vi "bigcryo_H-full_ver2.vi"() -> ()   [LabVIEW 2019]
uses:
  B_Globals.vi
  <vilib>/Analysis/NI_AALPro.lvlib
panel:
  out "Stable":bool
  out "Act. Rate [T/min]":dbl
  out "Read Buffer":string="0"
  in  "stop":bool
  out "Its":i32
  out "Running Sequence":bool
  in  "Set Field":dbl
  in  "Rate":dbl=0.2
  in  "Go To":bool=TRUE
  out "Field [T]":dbl=10.348
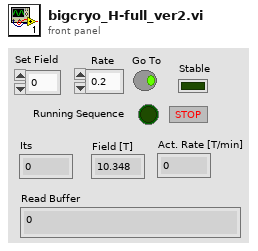
[diagram p1: front panel]
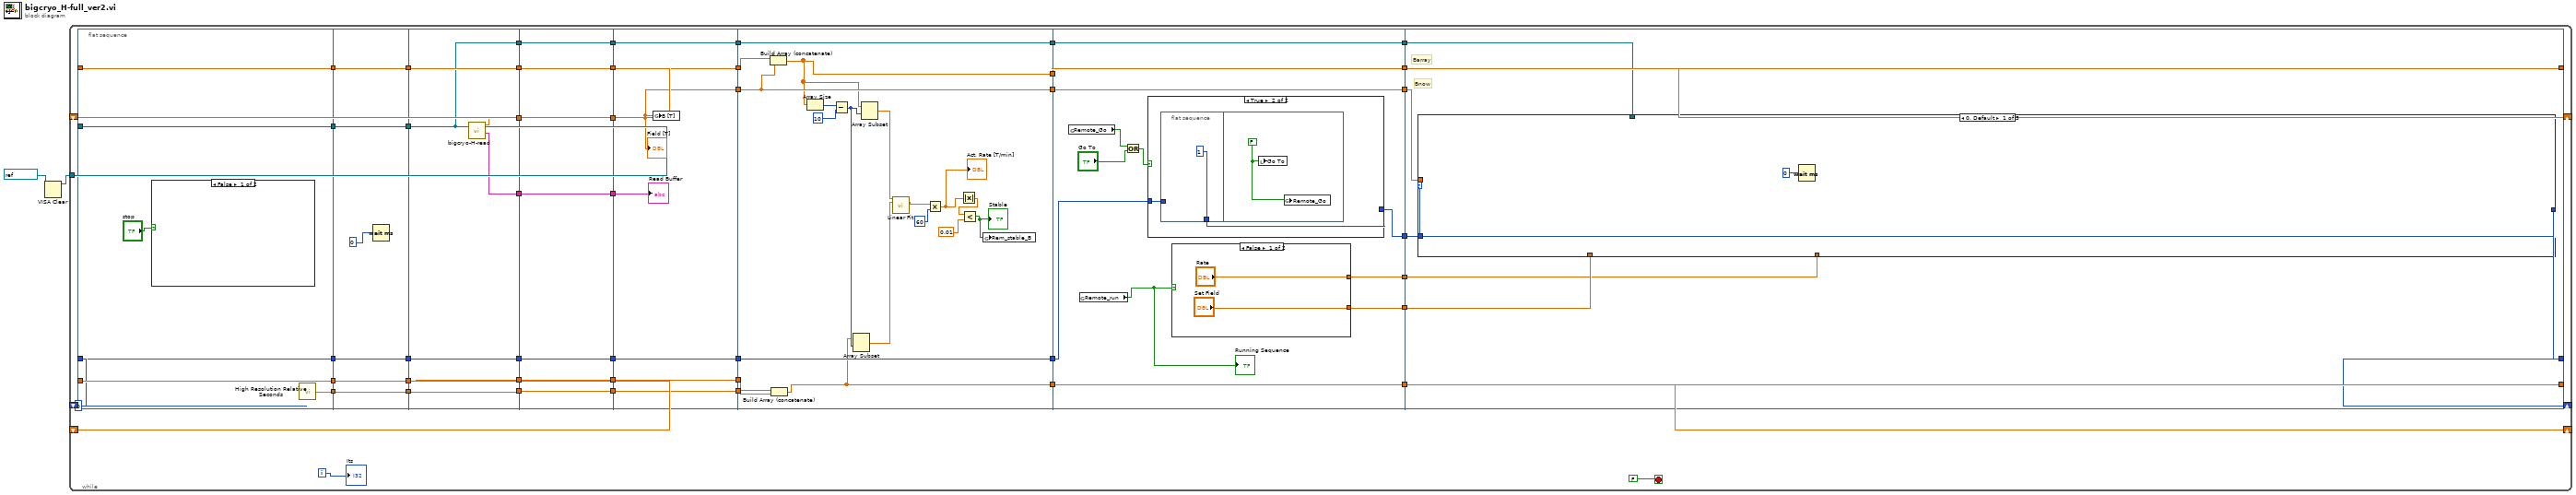
[diagram p0: block diagram]
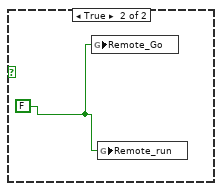
[diagram p2: hidden frame]
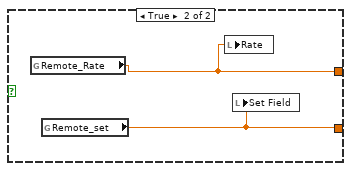
[diagram p3: hidden frame]
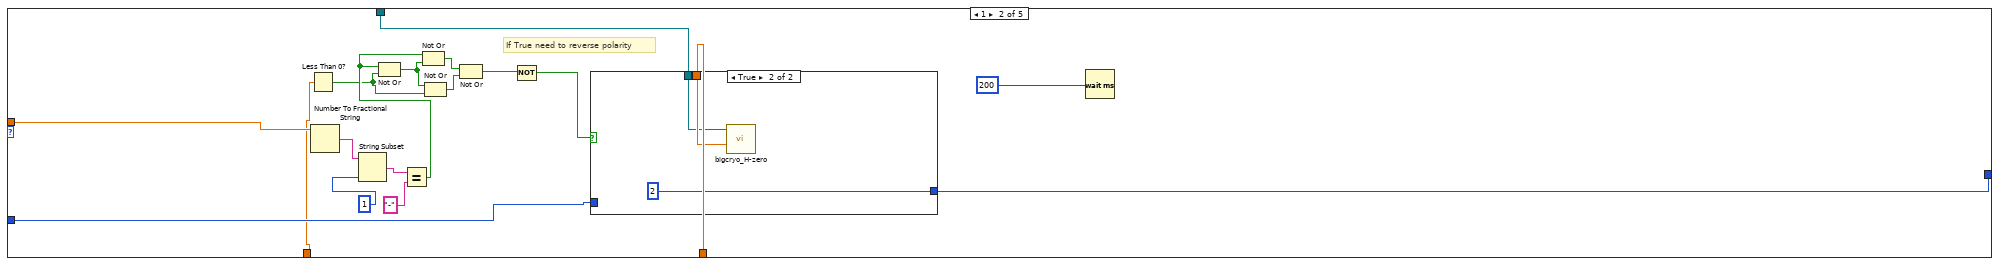
[diagram p5: hidden frame]
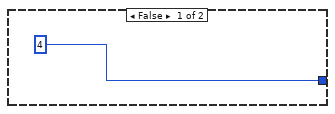
[diagram p6: hidden frame]
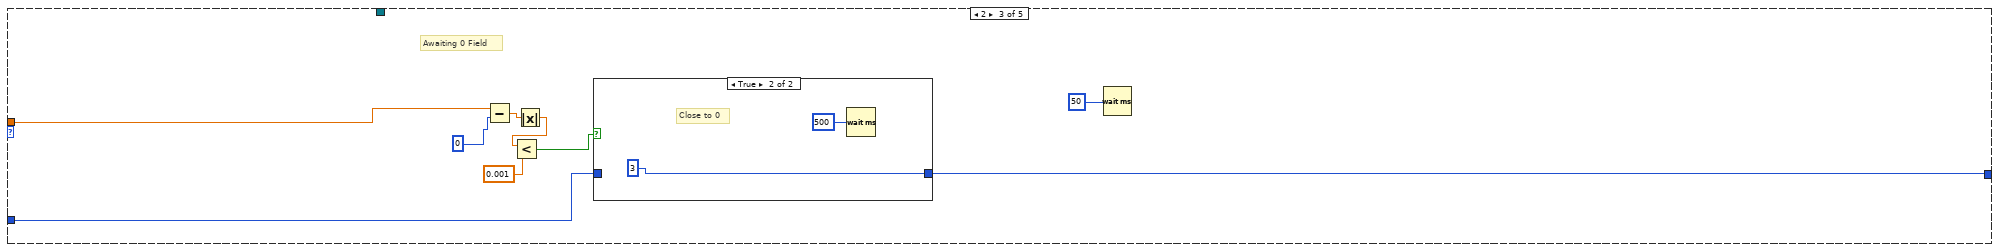
[diagram p7: hidden frame]
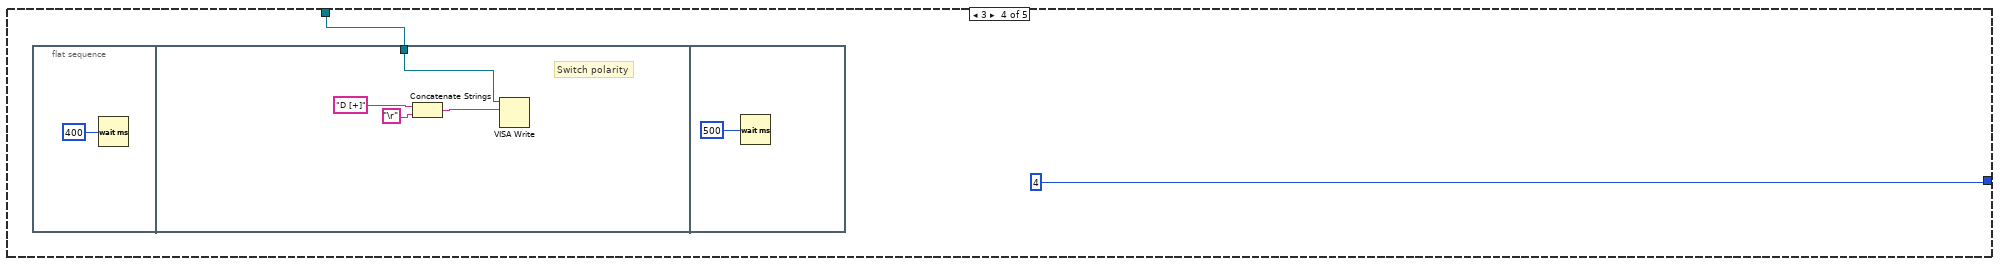
[diagram p9: hidden frame]
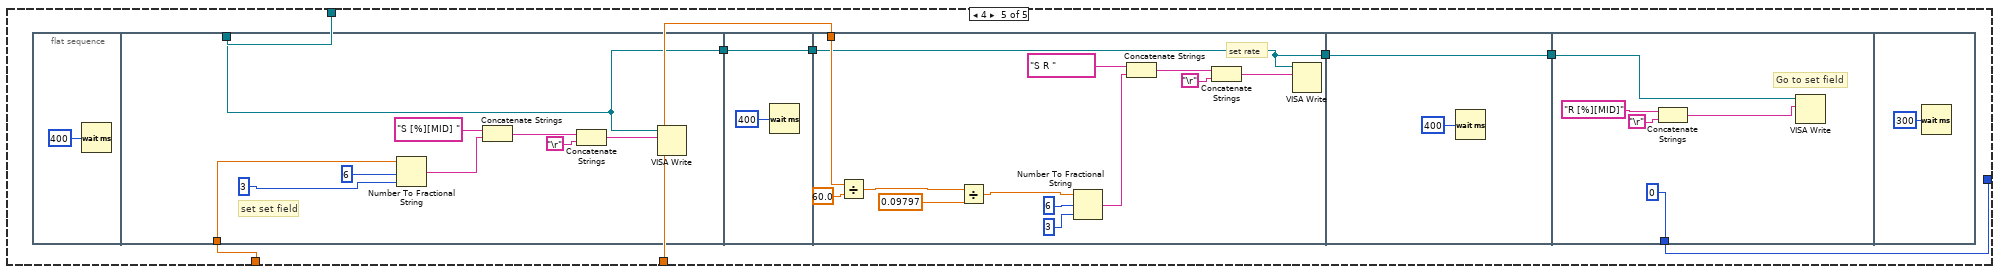
[diagram p10: hidden frame]
diagram:
  n1 = VISA Clear(VISA resource name=refnum<visa-resource-name> "COM6" ("Lakeshore Address")) -> (VISA resource name out=w2:refnum<visa-resource-name>)  [unwired: 1 in, 1 out]
  n2 = while {
    shift-right: [w52] -> _
    shift-left: _ -> [w53]
    shift-right: [w49] -> _
    shift-left: _ -> [w50]
    tunnel: w2 -> [w54]
    shift-right: [w40] -> _
    shift-left: 0 -> [w46]
    i -> [w31]
    stop <- FALSE stop-if-true
    n3 = flat-sequence {
      tunnel: w46 -> [w57]
      tunnel: w50 -> [w58]
      tunnel: w53 -> [w59]
      tunnel: w54 -> [w60]
      tunnel: [w60] -> w13
      tunnel: [w59] -> w11
      tunnel: [w58] -> w9
      tunnel: [w57] -> w7
      tunnel: [w55] -> w5
      tunnel: w13 -> [w67]
      tunnel: [w67] -> w12
      tunnel: w11 -> [w66]
      tunnel: [w66] -> w10
      tunnel: w9 -> [w65]
      tunnel: [w65] -> w8
      tunnel: w7 -> [w64]
      tunnel: [w64] -> w6
      tunnel: w5 -> [w63]
      tunnel: [w63] -> w4
      tunnel: [w74] -> w30
      tunnel: [w73] -> w28
      tunnel: [w72] -> w26
      tunnel: [w68] -> w24
      tunnel: [w71] -> w22
      tunnel: [w70] -> w20
      tunnel: w12 -> [w70]
      tunnel: w10 -> [w73]
      tunnel: w8 -> [w72]
      tunnel: w6 -> [w71]
      tunnel: [w69] -> w18
      tunnel: w4 -> [w68]
      tunnel: w30 -> [w81]
      tunnel: [w81] -> w29
      tunnel: w28 -> [w80]
      tunnel: [w80] -> w27
      tunnel: w26 -> [w79]
      tunnel: [w79] -> w25
      tunnel: w24 -> [w78]
      tunnel: [w78] -> w23
      tunnel: w22 -> [w77]
      tunnel: [w77] -> w21
      tunnel: w20 -> [w76]
      tunnel: [w76] -> w19
      tunnel: w18 -> [w75]
      tunnel: [w75] -> w17
      tunnel: w29 -> [w82]
      tunnel: w27 -> [w83]
      tunnel: w25 -> [w85]
      tunnel: w23 -> [w84]
      tunnel: w21 -> [w88]
      tunnel: [w88] -> w44
      tunnel: [w82] -> w37
      tunnel: w19 -> [w87]
      tunnel: [w87] -> w35
      tunnel: w17 -> [w86]
      tunnel: [w85] -> w16
      tunnel: [w84] -> w15
      tunnel: [w83] -> w14
      tunnel: [w99] -> w48
      tunnel: [w97] -> w47
      tunnel: [w107] -> w45
      tunnel: w44 -> [w107]
      tunnel: [w102] -> w38
      tunnel: w37 -> [w102]
      tunnel: [w106] -> w36
      tunnel: w35 -> [w106]
      tunnel: w16 -> [w105]
      tunnel: w15 -> [w104]
      tunnel: w14 -> [w103]
      tunnel: w48 -> [w119]
      tunnel: w47 -> [w118]
      tunnel: w45 -> [w114]
      tunnel: [w119] -> w43
      tunnel: [w118] -> w42
      tunnel: [w113] -> w41
      tunnel: [w112] -> w39
      tunnel: w38 -> [w112]
      tunnel: w36 -> [w111]
      tunnel: [w111] -> w34
      tunnel: [w109] -> w33
      tunnel: [w108] -> w32
      tunnel: [w135] -> w49
      tunnel: [w136] -> w52
      tunnel: w43 -> [w136]
      tunnel: w42 -> [w135]
      tunnel: w41 -> [w129]
      tunnel: [w134] -> w40
      tunnel: w39 -> [w133]
      tunnel: w34 -> [w132]
      tunnel: w33 -> [w131]
      tunnel: w32 -> [w130]
      frame #0 {
        n4 = case shown="False" "stop" {
          frame False {
          }
          frame True {
            w61 = FALSE
            n5 = global write "B_Globals.vi" "Remote_Go"(w61) -> ()
            n6 = global write "B_Globals.vi" "Remote_run"(w61) -> ()
          }
        }
        n7 = call <vilib>:"High Resolution Relative Seconds.vi"() -> ("relative seconds"=w55:dbl)
      }
      frame #1 {
        n8 = Wait (ms)(milliseconds to wait=u32 0 ("Pre Delay")) -> ()  [unwired: 1 out]
      }
      frame #2 {
        n9 = call "bigcryo-H-read.vi"("Magnet Power supply"=w70) -> ("substring"=w69:string, "Magnetic Field [T]"=w74:dbl)  [unwired: 9 in]
      }
      frame #3 {
      }
      frame #4 {
        n10 = global write "B_Globals.vi" "B [T]"(w82) -> ()
        "Field [T]" <- w82
        "Read Buffer" <- w86
      }
      frame #5 {
        n11 = Build Array (concatenate)(w103, w102) -> (w99:dbl[])
        n12 = Build Array (concatenate)(w105, w104) -> (w97:dbl[])
        n13 = Array Size(array=w99) -> (size(s)=w100:i32)
        n14 = Subtract(x=w100, y=10) -> (x-y=w98:i32)
        n15 = Array Subset(array=w97, index=w98) -> (w95:dbl[])  [unwired: 1 in]
        n16 = Array Subset(array=w99, index=w98) -> (w96:dbl[])  [unwired: 1 in]
        n17 = call <vilib>:"Linear Fit.vi"("Y"=w96, "X"=w95) -> ("slope"=w91:dbl)  [unwired: 9 in, 4 out]
        n18 = Multiply(x=w91, y=60) -> (x*y=w90:dbl)
        "Act. Rate [T/min]" <- w90
        n19 = Absolute Value(x=w90) -> (abs(x)=w92:dbl)
        n20 = Less?(x=w92, y=0.01) -> (x < y?=w89:bool)
        "Stable" <- w89
        n21 = global write "B_Globals.vi" "Rem_stable_B"(w89) -> ()
      }
      frame #6 {
        n22 = global read "B_Globals.vi" "Remote_Go"() -> (w117:bool)
        n23 = global read "B_Globals.vi" "Remote_run"() -> (w110:bool)
        "Running Sequence" <- w110
        n24 = Or(x=w117, y="Go To") -> (x .or. y?=w115:bool)
        n25 = case shown="True" w115 {
          tunnel: w114 -> [w124 w126]
          tunnel: [w124 w125] -> w113
          frame False {
          }
          frame True {
            n26 = flat-sequence {
              tunnel: w126 -> [_]
              tunnel: [1] -> w125
              frame #0 {
              }
              frame #1 {
                w128 = FALSE
                n27 = local write "Go To"(w128) -> ()
                n28 = global write "B_Globals.vi" "Remote_Go"(w128) -> ()
              }
            }
          }
        }
        n29 = case shown="False" w110 {
          tunnel: ["Set Field" w122] -> w109
          tunnel: ["Rate" w123] -> w108
          frame False {
          }
          frame True {
            n30 = global read "B_Globals.vi" "Remote_Rate"() -> (w123:dbl)
            n31 = global read "B_Globals.vi" "Remote_set"() -> (w122:dbl)
            n32 = local write "Rate"(w123) -> ()
            n33 = local write "Set Field"(w122) -> ()
          }
        }
      }
      frame #7 {
        # "Bnow"
        # "Barray"
        n34 = case shown="0, Default" w129 {
          tunnel: w133 -> [_ w152 w166 _ _]
          tunnel: w129 -> [w138 w145 w163 _ _]
          tunnel: [w138 w144 w162 4 w182] -> w134
          tunnel: w130 -> [_ w142 _ _ w185]
          tunnel: w132 -> [_ w141 _ w174 w188]
          tunnel: w131 -> [_ w139 _ _ w181]
          frame 0, Default {
            n35 = Wait (ms)(milliseconds to wait=0) -> ()  [unwired: 1 out]
          }
          frame 1 {
            # "If True need to reverse polarity"
            n36 = Less Than 0?(x=w139) -> (x < 0?=w143:bool)
            n37 = Number To Fractional String(number=w152) -> (F-format string=w155:string)  [unwired: 3 in]
            n38 = String Subset(string=w155, length (rest)=1 ("length (rest)")) -> (substring=w154:string)  [unwired: 1 in]
            n39 = Equal?(x=w154, y="-") -> (x = y?=w147:bool)
            n40 = Not Or(1:w143, 2:w147) -> (0:w151:bool)
            n41 = Not Or(1:w151, 2:w147) -> (0:w150:bool)
            n42 = Not Or(1:w143, 2:w151) -> (0:w149:bool)
            n43 = Not Or(1:w149, 2:w150) -> (0:w148:bool)
            n44 = Not(x=w148) -> (.not. x?=w146:bool)
            n45 = case shown="True" w146 {
              tunnel: w145 -> [_ _]
              tunnel: [4 2] -> w144
              tunnel: w142 -> [_ w159]
              tunnel: w141 -> [_ w158]
              frame False {
              }
              frame True {
                n46 = call "bigcryo_H-zero.vi"("Rate [T/min]"=w159, "Magnet Power supply"=w158) -> ()  [unwired: 10 in]
              }
            }
            n47 = Wait (ms)(milliseconds to wait=200) -> ()  [unwired: 1 out]
          }
          frame 2 {
            # "Awaiting 0 Field"
            n48 = Subtract(x=w166, y=0) -> (x-y=w168:dbl)
            n49 = Absolute Value(x=w168) -> (abs(x)=w165:dbl)
            n50 = Less?(x=w165, y=0.001) -> (x < y?=w164:bool)
            n51 = case shown="True" w164 {
              tunnel: w163 -> [w170 _]
              tunnel: [w170 3] -> w162
              frame False {
              }
              frame True {
                # "Close to 0"
                n52 = Wait (ms)(milliseconds to wait=500) -> ()  [unwired: 1 out]
              }
            }
            n53 = Wait (ms)(milliseconds to wait=50) -> ()  [unwired: 1 out]
          }
          frame 3 {
            n54 = flat-sequence {
              tunnel: w174 -> [w176]
              frame #0 {
                n55 = Wait (ms)(milliseconds to wait=400) -> ()  [unwired: 1 out]
              }
              frame #1 {
                # "Switch polarity"
                n56 = Concatenate Strings("D [+]" ("data"), "\r") -> (w179:string)
                n57 = VISA Write(VISA resource name=w176, write buffer=w179) -> ()  [unwired: 1 in, 3 out]
              }
              frame #2 {
                n58 = Wait (ms)(milliseconds to wait=500) -> ()  [unwired: 1 out]
              }
            }
          }
          frame 4 {
            n59 = flat-sequence {
              tunnel: w188 -> [w191]
              tunnel: [w191] -> w186
              tunnel: w181 -> [w190]
              tunnel: [w199] -> w187
              tunnel: w186 -> [w199]
              tunnel: w187 -> [w201]
              tunnel: w185 -> [w202]
              tunnel: [w201] -> w183
              tunnel: [w215] -> w184
              tunnel: w183 -> [w215]
              tunnel: w184 -> [w217]
              tunnel: [0] -> w182
              frame #0 {
                n60 = Wait (ms)(milliseconds to wait=400) -> ()  [unwired: 1 out]
              }
              frame #1 {
                # "set set field"
                n61 = Number To Fractional String(number=w190, width (-)=i16 6, precision (6)=i16 3) -> (F-format string=w195:string)  [unwired: 1 in]
                n62 = Concatenate Strings("S [%][MID] " ("string"), w195) -> (w192:string)
                n63 = Concatenate Strings(w192, "\r") -> (w194:string)
                n64 = VISA Write(VISA resource name=w191, write buffer=w194) -> ()  [unwired: 1 in, 3 out]
              }
              frame #2 {
                n65 = Wait (ms)(milliseconds to wait=400) -> ()  [unwired: 1 out]
              }
              frame #3 {
                # "set rate"
                n66 = Divide(x=w202, y=60.0) -> (x/y=w207:dbl)
                n67 = Divide(x=w207, y=0.09797) -> (x/y=w205:dbl)
                n68 = Number To Fractional String(number=w205, width (-)=i16 6, precision (6)=i16 3) -> (F-format string=w210:string)  [unwired: 1 in]
                n69 = Concatenate Strings("S R " ("string"), w210) -> (w209:string)
                n70 = Concatenate Strings(w209, "\r") -> (w213:string)
                n71 = VISA Write(VISA resource name=w201, write buffer=w213) -> ()  [unwired: 1 in, 3 out]
              }
              frame #4 {
                n72 = Wait (ms)(milliseconds to wait=400) -> ()  [unwired: 1 out]
              }
              frame #5 {
                # "Go to set field"
                n73 = Concatenate Strings("R [%][MID]" ("data"), "\r") -> (w220:string)
                n74 = VISA Write(VISA resource name=w217, write buffer=w220) -> ()  [unwired: 1 in, 3 out]
              }
              frame #6 {
                n75 = Wait (ms)(milliseconds to wait=300) -> ()  [unwired: 1 out]
              }
            }
          }
        }
      }
    }
    "Its" <- w31
  }
